vi "Shutdown.vi"(8 "error in":errorcluster, 11 "FunctionGenerator in":refnum<class "FunctionGenerator.lvclass">) -> (0 "error out":errorcluster, 3 "FunctionGenerator out":refnum<class "FunctionGenerator.lvclass">)   [LabVIEW 2019, in "FunctionGenerator.lvlib" / "FunctionGenerator.lvclass"]
uses:
  Library/FunctionGenerator.lvclass
  builds/Instruments/Instruments.lvlibp/Library/Instruments.lvclass
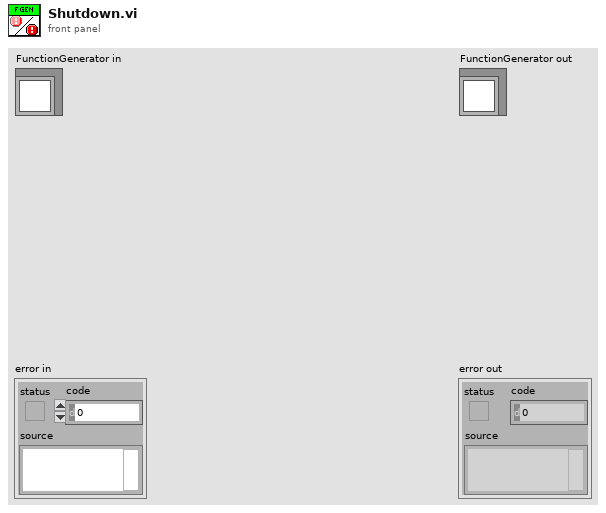
[diagram p1: front panel]
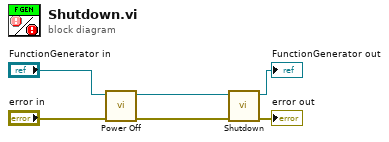
[diagram p0: block diagram]
diagram:
  n1 = call-dynamic "Power Off.vi"("error in (no error)"="error in", "FunctionGenerator in"="FunctionGenerator in") -> ("error out"=w2:errorcluster, "FunctionGenerator out"=w1:refnum<class "FunctionGenerator.lvclass">)  [unwired: 8 in]
  n2 = call-parent "Shutdown.vi"("error in"=w2, "Instruments in"=w1) -> ("error out"=→"error out":errorcluster, "Instruments out"=→"FunctionGenerator out":refnum<class "FunctionGenerator.lvclass">)  [unwired: 8 in]
